vi "Draw Tray Status.vi"() -> ()   [LabVIEW 2019]
panel:
  out "Image":T1(plugin-control)
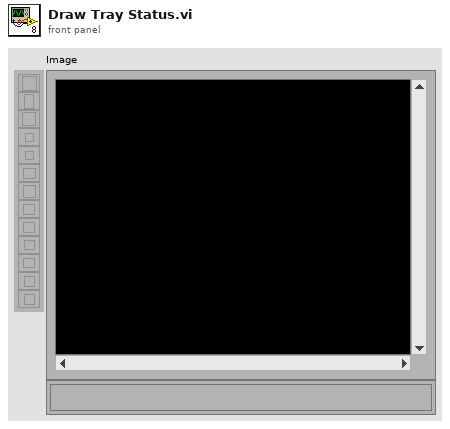
[diagram p1: front panel]
types:
  T1 = typedef "IMAQ Image.ctl" = refnum<image>
  T2 = cluster{"Left":i32, "Top":i32, "Right":i32, "Bottom":i32}
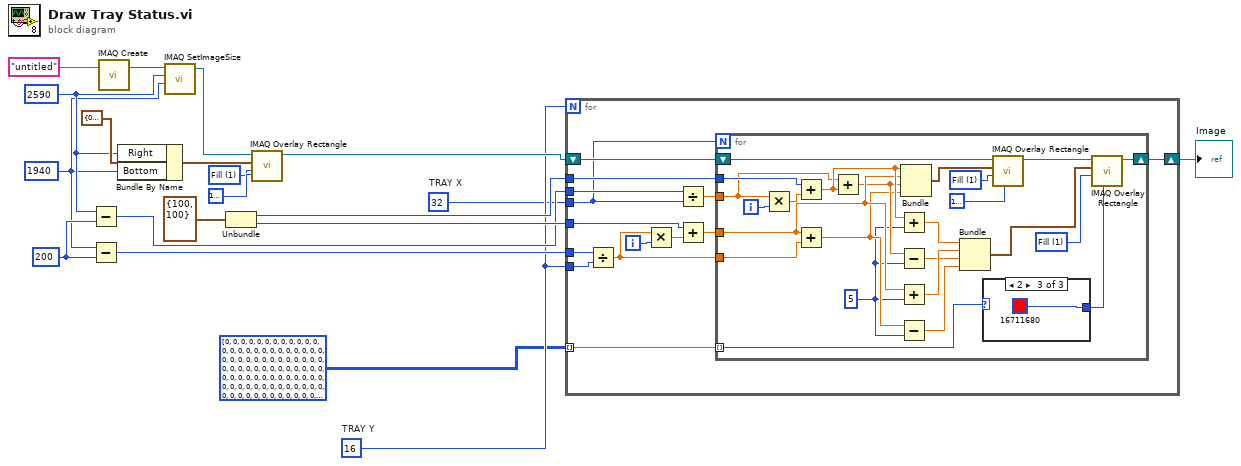
[diagram p0: block diagram]
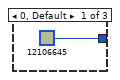
[diagram p2: hidden frame]
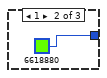
[diagram p3: hidden frame]
diagram:
  w2 = 32  # TRAY X
  w10 = 200 ("y")
  w11 = u32 1 items=["Frame", "Fill", "Highlight"] ("Drawing Mode (Frame)")
  w3 = 16  # TRAY Y
  w4 = 1940 ("X Resolution")
  w5 = 2590 ("X Resolution")
  n1 = Subtract(x=w5, y=w10) -> (x-y=w9:i32)
  n2 = Subtract(x=w4, y=w10) -> (x-y=w8:i32)
  n3 = call "IMAQ Create"("Image Name"="untitled") -> ("New Image"=w19:T1)  [unwired: 4 in, 1 out]
  n4 = Bundle By Name(cluster=T2 {"Left"=0, "Top"=0, "Right"=1280, "Bottom"=1400} ("Rectangle"), "Right"=w5, "Bottom"=w4) -> (w6:T2)
  n5 = call "IMAQ SetImageSize"("Y Resolution"=w4, "X Resolution"=w5, "Image"=w19) -> ("Image Out"=w18:T1)  [unwired: 2 in, 1 out]
  n6 = Unbundle(cluster{"Left":i32, "Top":i32} {"Left"=100, "Top"=100} ("Rectangle")) -> ("Left"=w14:i32, "Top"=w13:i32)
  n7 = call "IMAQ Overlay Rectangle"("Color"=u32 16777225, "Drawing Mode (Frame)"=w11, "Rectangle"=w6, "Image"=w18) -> ("Image Out"=w17:T1)  [unwired: 6 in, 1 out]
  n8 = for {
    N: w3 -> [_]
    shift-right: [w33] -> w16
    shift-left: w17 -> [w34]
    tunnel: w14 -> [w31]
    tunnel: w13 -> [w30]
    tunnel: w9 -> [w25]
    tunnel: w8 -> [w24]
    tunnel: w3 -> [w26]
    tunnel: w2 -> [w22]
    tunnel: i32[][] [[0, 0, 0, 0, 0, 0, 0, 0, 0, 0, 0, 0, 0, 0, 0, 0, 0, 0, 0, 0, 0, 0, 0, 0, 0, 0, 0, 0, 0, 0, 0, 0, 0], [0, 0, 0, 0, 0, 0, 0, 0, 0, 0, 0, 0, 0, 0, 0, 0, 0, 0, 0, 0, 0, 0, 0, 0, 0, 0, 0, 0, 0, 0, 0, 0, 0], [0, 0, 0, 0, 0, 0, 0, 0, 0, 0, 0, 0, 0, 0, 0, 0, 0, 0, 0, 0, 0, 0, 0, 0, 0, 0, 0, 0, 0, 0, 0, 0, 0], [0, 0, 0, 0, 0, 0, 0, 0, 0, 0, 0, 0, 0, 0, 0, 0, 0, 0, 0, 0, 0, 0, 0, 0, 0, 0, 0, 0, 0, 0, 0, 0, 0], [0, 0, 0, 0, 0, 0, 0, 0, 0, 0, 0, 0, 0, 0, 0, 0, 0, 0, 0, 0, 0, 0, 0, 0, 0, 0, 0, 0, 0, 0, 0, 0, 0], [0, 0, 0, 0, 0, 0, 0, 0, 0, 0, 0, 0, 0, 0, 0, 0, 0, 0, 0, 0, 0, 0, 0, 0, 0, 0, 0, 0, 0, 0, 0, 0, 0], [0, 0, 0, 0, 0, 0, 0, 0, 0, 0, 0, 0, 0, 0, 0, 0, 0, 0, 0, 0, 0, 0, 0, 0, 0, 0, 0, 0, 0, 0, 0, 0, 0], [0, 0, 0, 0, 0, 0, 0, 0, 0, 0, 0, 0, 0, 0, 0, 0, 0, 0, 0, 0, 0, 0, 0, 0, 0, 0, 0, 0, 0, 0, 0, 0, 0], [0, 0, 0, 0, 0, 0, 0, 0, 0, 0, 0, 0, 0, 0, 0, 0, 0, 0, 0, 0, 0, 0, 0, 0, 0, 0, 0, 0, 0, 0, 0, 0, 0], [0, 0, 0, 0, 0, 0, 0, 0, 0, 0, 0, 0, 0, 0, 0, 0, 0, 0, 0, 0, 0, 0, 0, 0, 0, 0, 0, 0, 0, 0, 0, 0, 0], [0, 0, 0, 0, 0, 0, 0, 0, 0, 0, 0, 0, 0, 0, 0, 0, 0, 0, 0, 0, 0, 0, 0, 0, 0, 0, 0, 0, 0, 0, 0, 0, 0], [0, 0, 0, 0, 0, 0, 0, 0, 0, 0, 0, 0, 0, 0, 0, 0, 0, 0, 0, 0, 0, 0, 0, 0, 0, 0, 0, 0, 0, 0, 0, 0, 0], [0, 0, 0, 0, 0, 0, 0, 0, 0, 0, 0, 0, 0, 0, 0, 0, 0, 0, 0, 0, 0, 0, 0, 0, 0, 0, 0, 0, 0, 0, 0, 0, 0], [0, 0, 0, 0, 0, 0, 0, 0, 0, 0, 0, 0, 0, 0, 0, 0, 0, 0, 0, 0, 0, 0, 0, 0, 0, 0, 0, 0, 0, 0, 0, 0, 0], [0, 0, 0, 0, 0, 0, 0, 0, 0, 0, 0, 0, 0, 0, 0, 0, 0, 0, 0, 0, 0, 0, 0, 0, 0, 0, 0, 0, 0, 0, 0, 0, 0], [0, 0, 0, 0, 0, 0, 0, 0, 0, 0, 0, 0, 0, 0, 0, 0, 0, 0, 0, 0, 0, 0, 0, 0, 0, 0, 0, 0, 0, 0, 0, 0, 0], [0, 0, 0, 0, 0, 0, 0, 0, 0, 0, 0, 0, 0, 0, 0, 0, 0, 0, 0, 0, 0, 0, 0, 0, 0, 0, 0, 0, 0, 0, 0, 0, 0]] -> [w21] mode=indexing
    i -> [w32]
    n9 = Divide(x=w24, y=w26) -> (x/y=w23:dbl)
    n10 = Multiply(x=w23, y=w32) -> (x*y=w29:dbl)
    n11 = Divide(x=w25, y=w22) -> (x/y=w27:dbl)
    n12 = Add(x=w30, y=w29) -> (x+y=w28:dbl)
    n13 = for {
      N: w22 -> [_]
      shift-right: [w57] -> w33
      shift-left: w34 -> [w51]
      tunnel: w31 -> [w55]
      tunnel: w28 -> [w47]
      tunnel: w27 -> [w38]
      tunnel: w23 -> [w37]
      tunnel: w21 -> [w36] mode=indexing
      i -> [w56]
      w44 = 5 ("y")
      w52 = u32 1 items=["Frame", "Fill", "Highlight"] ("Drawing Mode (Frame)")
      w58 = u32 1 items=["Frame", "Fill", "Highlight"] ("Drawing Mode (Frame)")
      n14 = Multiply(x=w38, y=w56) -> (x*y=w54:dbl)
      n15 = Add(x=w55, y=w54) -> (x+y=w48:dbl)
      n16 = Add(x=w47, y=w37) -> (x+y=w45:dbl)
      n17 = Add(x=w38, y=w48) -> (x+y=w46:dbl)
      n18 = Add(x=w48, y=w44) -> (x+y=w43:dbl)
      n19 = Subtract(x=w46, y=w44) -> (x-y=w41:dbl)
      n20 = Add(x=w47, y=w44) -> (x+y=w42:dbl)
      n21 = Subtract(x=w45, y=w44) -> (x-y=w40:dbl)
      n22 = Bundle(w48, w47, w46, w45) -> (w49:cluster{dbl, dbl, dbl, dbl})  [unwired: 1 in]
      n23 = Bundle(w43, w42, w41, w40) -> (w39:cluster{dbl, dbl, dbl, dbl})  [unwired: 1 in]
      n24 = case shown="2" w36 {
        tunnel: [u32 12106645 ("Color") u32 6618880 ("Color") u32 16711680 ("Color")] -> w35
        frame 0, Default {
        }
        frame 1 {
        }
        frame 2 {
        }
      }
      n25 = call "IMAQ Overlay Rectangle"("Color"=u32 16777228, "Drawing Mode (Frame)"=w52, "Rectangle"=w49, "Image"=w51) -> ("Image Out"=w50:T1)  [unwired: 6 in, 1 out]
      n26 = call "IMAQ Overlay Rectangle"("Color"=w35, "Drawing Mode (Frame)"=w58, "Rectangle"=w39, "Image"=w50) -> ("Image Out"=w57:T1)  [unwired: 6 in, 1 out]
    }
  }
  "Image" <- w16
